vi "AutoTurnToHotFromCenter.vi"(8 "error in (no error)":errorcluster, 10 "Left/Right":enum16{"Left", "Right", ""}(ring), 11 "Hot?":bool) -> (0 "error out":errorcluster)   [LabVIEW 2013]
uses:
  AutoTurnToHotStates.ctl
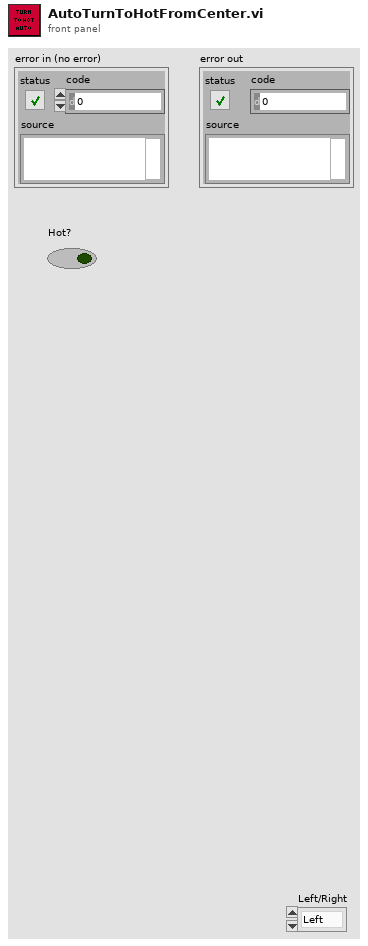
[diagram p1: front panel]
types:
  T1 = typedef "AutoTurnToHotStates.ctl" = enum16{"Wait For Pos", "Check Hot", "Turn", "Fire"}
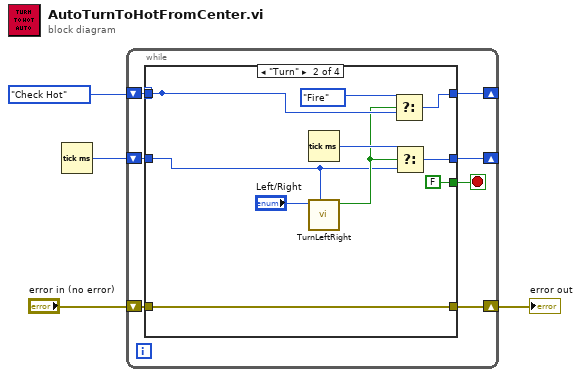
[diagram p0: block diagram]
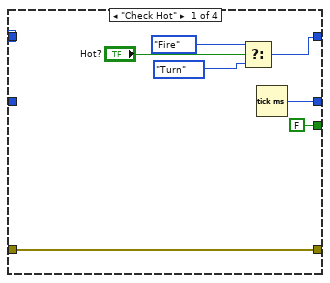
[diagram p2: hidden frame]
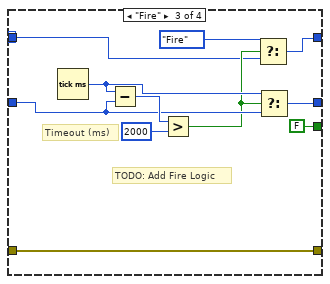
[diagram p3: hidden frame]
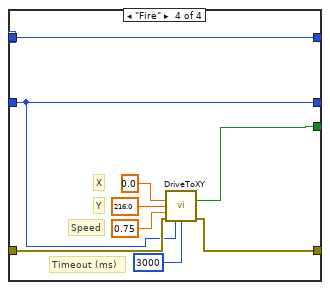
[diagram p4: hidden frame]
diagram:
  n1 = Tick Count (ms)() -> (millisecond timer value=w4:u32)
  n2 = while {
    shift-right: [w10] -> w3
    shift-left: "error in (no error)" -> [w11]
    shift-right: [w8] -> _
    shift-left: w4 -> [w9]
    shift-right: [w5] -> _
    shift-left: AutoTurnToHotStates."Check Hot" -> [w6]
    stop <- w7 stop-if-true
    n3 = case shown="\"Turn\"" w6 {
      selector: w6 -> [_ w26 w33 w40]
      tunnel: w11 -> [w14 w24 w31 w45]
      tunnel: [w14 w24 w31 w44] -> w10
      tunnel: [w17 w25 w32 w40] -> w5
      tunnel: w9 -> [_ w19 w36 w42]
      tunnel: [w16 w27 w34 w42] -> w8
      tunnel: [FALSE FALSE FALSE w41] -> w7
      tunnel: w6 -> [_ _ _ _]
      frame "Check Hot" {
        n4 = Select(t=AutoTurnToHotStates."Fire", s="Hot?", f=AutoTurnToHotStates."Turn") -> (s? t:f=w17:T1)
        n5 = Tick Count (ms)() -> (millisecond timer value=w16:u32)
      }
      frame "Turn" {
        n6 = Tick Count (ms)() -> (millisecond timer value=w28:u32)
        n7 = call "TurnLeftRight.vi"("Start time"=w19, "Left/Right"="Left/Right") -> ("Done"=w20:bool)  [unwired: 9 in]
        n8 = Select(t=AutoTurnToHotStates."Fire", s=w20, f=w26) -> (s? t:f=w25:T1)
        n9 = Select(t=w28, s=w20, f=w19) -> (s? t:f=w27:u32)
      }
      frame "Fire" {
        # "TODO: Add Fire Logic"
        # "Timeout (ms)"
        n10 = Tick Count (ms)() -> (millisecond timer value=w39:u32)
        n11 = Subtract(x=w39, y=w36) -> (x-y=w38:u32)
        n12 = Greater?(x=w38, y=u32 2000) -> (0:w35:bool)
        n13 = Select(t=AutoTurnToHotStates."Fire", s=w35, f=w33) -> (s? t:f=w32:T1)
        n14 = Select(t=w39, s=w35, f=w36) -> (s? t:f=w34:u32)
      }
      frame "Fire" {
        # "Timeout (ms)"
        # "Speed"
        # "Y"
        # "X"
        n15 = call "DriveToXY.vi"("X Target"=0.0, "Y Target"=216.0, "Speed"=0.75, "error in"=w45, "Start time"=w42, "Timeout (ms)"=u32 3000 ("y")) -> ("At Target"=w41:bool, "error out"=w44:errorcluster)  [unwired: 6 in, 2 out]
      }
    }
  }
  "error out" <- w3
